vi "changeDigitalFilter.vi"(8 "error in (no error)":errorcluster, 10 "ElectrometerController in":refnum<class "ElectrometerController.lvclass">, 11 "State in":refnum<class "ElectrometerState.lvclass">) -> (0 "error out":errorcluster, 2 "ElectrometerController out":refnum<class "ElectrometerController.lvclass">, 3 "State out":refnum<class "ElectrometerState.lvclass">)   [LabVIEW 2016, in "ElectrometerState.lvclass"]
uses:
  ElectrometerState.lvclass
  ElectrometerController/ElectrometerController.lvclass
  ts_electrometeruserevents/Typedefs/RejectedCommand.ctl
  ts_electrometeruserevents/Typedefs/CommandValue.ctl
  ts_electrometeruserevents/Typedefs/StateValue.ctl
  ts_electrometeruserevents/Typedefs/ElectrometerTypedefs.lvlib
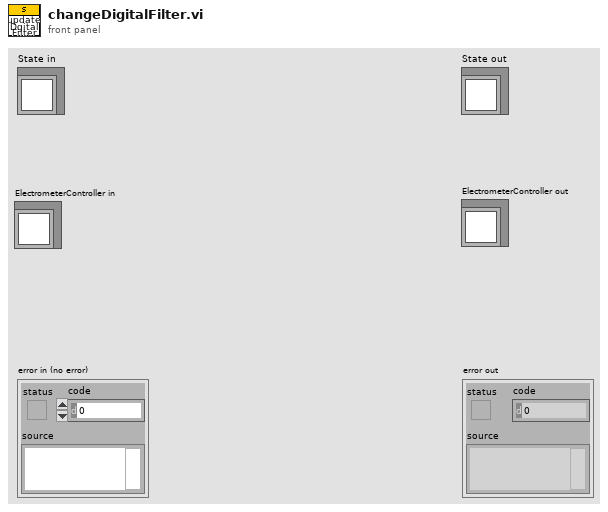
[diagram p1: front panel]
types:
  T1 = typedef "ElectrometerTypedefs.lvlib/RejectedCommand.ctl" = cluster{"CommandValue":T2, "StateValue":T3, "Time Stamp":dbl}
  T2 = typedef "ElectrometerTypedefs.lvlib/CommandValue.ctl" = enum16{"ClearError", "Disable", "Enable", "Exit", "GoToStandby", "OnHeartbeat", "OnIncomingMessagingError", "OnInterrupt", "Start", "SetDigitalFilter", "StartScan", "StartScanDt", "StartScanReachIntensity", "StopScan", "SetIntegrationTime", "PerformZeroCalib", "SetRange", "SetMode", "Power"}
  T3 = typedef "ElectrometerTypedefs.lvlib/StateValue.ctl" = enum16{"OffState", "StandbyState", "DisabledState", "EnabledState", "FaultState", "SetDurationReadingState", "ConfiguringState", "ReadyState", "ManualReadingState", "UntilIntentisyReadingState"}
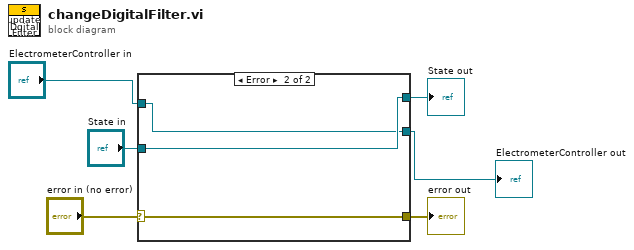
[diagram p0: block diagram]
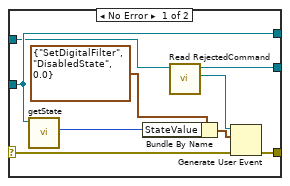
[diagram p2: hidden frame]
diagram:
  n1 = case shown="Error" "error in (no error)" {
    selector: "error in (no error)" -> [w12 w18]
    tunnel: [w11 w18] -> w5
    tunnel: [w10 w17] -> w3
    tunnel: "State in" -> [w10 w17]
    tunnel: "ElectrometerController in" -> [w9 w16]
    tunnel: [w7 w16] -> w1
    frame No Error {
      n2 = call-dynamic "getState.vi"("State in"=w10) -> ("StateValue"=w13:T3)  [unwired: 8 in, 2 out]
      n3 = Bundle By Name(cluster=T1 {"CommandValue"=enum."SetDigitalFilter", "StateValue"=enum."DisabledState", "Time Stamp"=0.0} ("event data"), "StateValue"=w13) -> (w14:T1)
      n4 = call-dynamic "Read RejectedCommand.vi"("ElectrometerController in"=w9) -> ("RejectedCommand"=w8:refnum<user-event>, "ElectrometerController out"=w7:refnum<class "ElectrometerController.lvclass">)  [unwired: 8 in, 1 out]
      n5 = Generate User Event(user event=w8, event data cluster=w14, error in=w12) -> (error out=w11:errorcluster)  [unwired: 1 in, 1 out]
    }
    frame Error {
    }
  }
  "error out" <- w5
  "State out" <- w3
  "ElectrometerController out" <- w1
